vi "Actor Core.vi"(8 "error in":errorcluster, 11 "PAS Actor in":refnum<class "PAS Actor.lvclass">) -> (0 "error out":errorcluster, 3 "Actor out":refnum<class "Actor.lvclass">)   [LabVIEW 2013, in "PAS Actor.lvclass"]
doc: "(<B>Filename</B>: Actor Framework.lvlib:Actor.lvclass:Actor Core.vi)\n\nReceives messages to the actor, reacts to them, and initiates any error handling that may shut the actor down.\n\nDescendant classes may override this VI to append parallel tasks for the actor to complete while it handles messages. Overrides use the Call Parent Method node."
uses:
  PAS Actor.lvclass
  <vilib>/ActorFramework/Actor/Actor.lvclass
  PAS Actor.lvclass/PAS Actor.ctl
  <vilib>/Utility/error.llb/DialogType.ctl
  Main/PAS.lvclass
  Instrument/state.ctl
  Commands/Command.lvclass
  Instrument/Instrument.lvclass
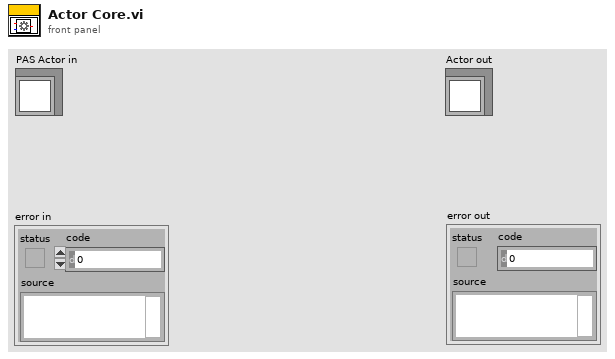
[diagram p1: front panel]
types:
  T1 = typedef "Instrument.lvclass/state.ctl" = enum8{"Configure", "Acquire", "Wait", "Quit", "Handle Error", "NOOP"}
  T2 = typedef "DialogType.ctl" = u16
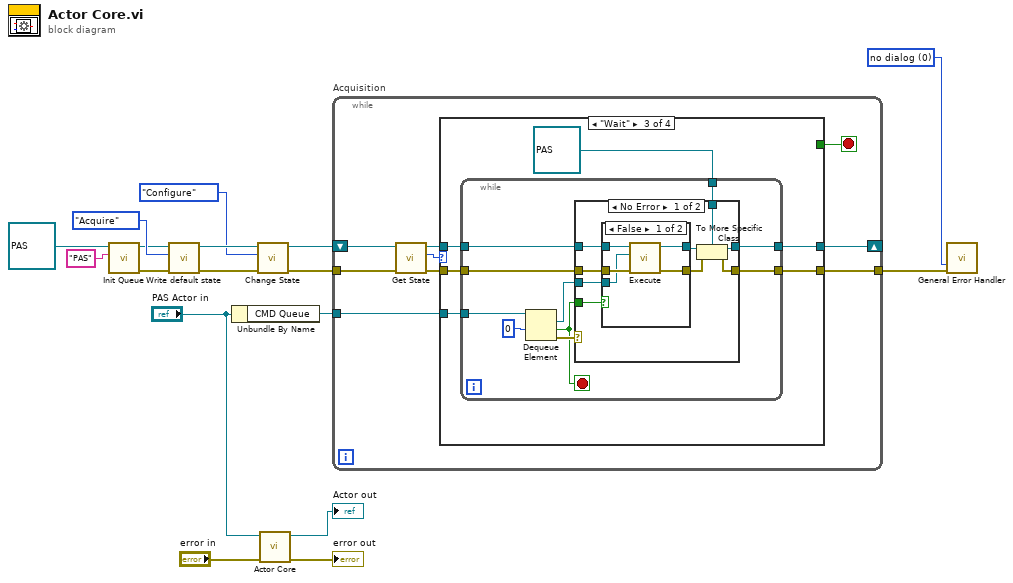
[diagram p0: block diagram]
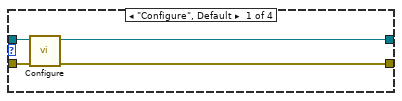
[diagram p2: hidden frame]
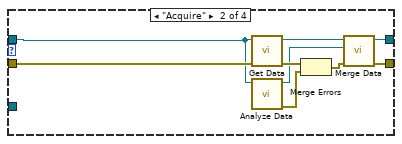
[diagram p3: hidden frame]
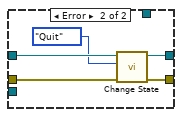
[diagram p5: hidden frame]
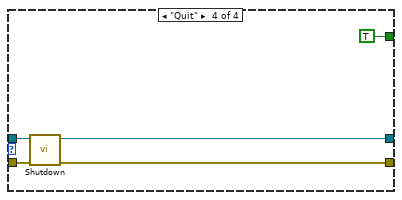
[diagram p6: hidden frame]
diagram:
  w13 = T2 0 items=["no dialog", "OK message", "continue or stop message", "OK message + warnings", "continue/stop + warnings"] ("type of dialog (OK msg:1)")
  n1 = call "Init Queue.vi"("queue_name"="PAS", "Instrument in"=refnum<class "PAS.lvclass"> refnum ("PAS")) -> ("error out"=w3:errorcluster, "Instrument out"=w4:refnum<class "PAS.lvclass">)  [unwired: 8 in]
  n2 = call "Write default state.vi"("error in (no error)"=w3, "instr state"=state."Acquire", "Instrument in"=w4) -> ("error out"=w6:errorcluster, "Instrument out"=w7:refnum<class "PAS.lvclass">)  [unwired: 7 in]
  n3 = Unbundle By Name("PAS Actor in") -> ("CMD Queue"=w11:refnum<queue>)
  n4 = call "Change State.vi"("error in"=w6, "instr state"=state."Configure", "Instrument in"=w7) -> ("error out"=w8:errorcluster, "Instrument out"=w9:refnum<class "PAS.lvclass">)  [unwired: 7 in]
  n5 = call-parent "Actor Core.vi"("error in"="error in", "Actor in"="PAS Actor in") -> ("error out"=→"error out":errorcluster, "Actor out"=→"Actor out":refnum<class "Actor.lvclass">)  [unwired: 8 in]
  n6 = while "Acquisition" {
    tunnel: w8 -> [w26]
    shift-right: [w20] -> _
    shift-left: w9 -> [w24]
    tunnel: [w19] -> w14
    tunnel: w11 -> [w18]
    stop <- w21 stop-if-true
    n7 = call "Get State.vi"("error in"=w26, "Instrument in"=w24) -> ("error out"=w22:errorcluster, "default state"=w25:T1, "Instrument out"=w23:refnum<class "PAS.lvclass">)  [unwired: 7 in]
    n8 = case shown="\"Wait\"" w25 {
      tunnel: w23 -> [w30 w38 w44 w80]
      tunnel: w22 -> [w29 w39 w42 w79]
      tunnel: [_ _ _ TRUE] -> w21
      tunnel: [w28 w34 w43 w78] -> w20
      tunnel: [w27 w32 w41 w77] -> w19
      tunnel: w18 -> [_ _ w45 _]
      frame "Configure", Default {
        n9 = call-dynamic "Configure.vi"("error in"=w29, "PAS in"=w30) -> ("error out"=w27:errorcluster, "PAS out"=w28:refnum<class "PAS.lvclass">)  [unwired: 8 in]
      }
      frame "Acquire" {
        n10 = call-dynamic "Get Data.vi"("error in"=w39, "PAS in"=w38) -> ("error out"=w37:errorcluster, "PAS out"=w35:refnum<class "PAS.lvclass">)  [unwired: 8 in]
        n11 = call-dynamic "Analyze Data.vi"("PAS in"=w38) -> ("error out"=w36:errorcluster, "PAS out"=w31:refnum<class "PAS.lvclass">)  [unwired: 9 in]
        n12 = Merge Errors(w37, w36) -> (w33:errorcluster)
        n13 = call-dynamic "Merge Data.vi"("error in"=w33, "Analyzed"=w31, "Acquired"=w35) -> ("error out"=w32:errorcluster, "PAS out"=w34:refnum<class "PAS.lvclass">)  [unwired: 7 in]
      }
      frame "Wait" {
        n14 = while {
          tunnel: w45 -> [w55]
          tunnel: w44 -> [w54]
          tunnel: [w53] -> w43
          tunnel: w42 -> [w52]
          tunnel: [w51] -> w41
          tunnel: refnum<class "PAS.lvclass"> refnum ("PAS") -> [w46]
          stop <- w48 stop-if-true
          n15 = Dequeue Element(queue=w55, timeout in ms (-1)=0) -> (element=w47:refnum<class "Command.lvclass">, timed out?=w48:bool, error out=w49:errorcluster)  [unwired: 1 in, 1 out]
          n16 = case shown="No Error" w49 {
            tunnel: w54 -> [w64 w76]
            tunnel: [w58 w74] -> w53
            tunnel: w52 -> [w63 w75]
            tunnel: [w56 w73] -> w51
            tunnel: w48 -> [w62 _]
            tunnel: w47 -> [w61 _]
            tunnel: w46 -> [w57 _]
            frame No Error {
              n17 = case shown="False" w62 {
                tunnel: w64 -> [w69 w71]
                tunnel: [w68 w71] -> w59
                tunnel: w63 -> [w67 w70]
                tunnel: [w66 w70] -> w60
                tunnel: w61 -> [w65 _]
                frame False {
                  n18 = call-dynamic "Execute.vi"("error in"=w67, "Command in"=w65, "Instrument In"=w69) -> ("error out"=w66:errorcluster, "Instrument Out"=w68:refnum<class "Instrument.lvclass">)  [unwired: 7 in]
                }
                frame True {
                }
              }
              n19 = To More Specific Class(target class=w57, reference=w59, error in=w60) -> (specific class reference=w58:refnum<class "PAS.lvclass">, error out=w56:errorcluster)
            }
            frame Error {
              n20 = call "Change State.vi"("error in"=w75, "instr state"=state."Quit", "Instrument in"=w76) -> ("error out"=w73:errorcluster, "Instrument out"=w74:refnum<class "PAS.lvclass">)  [unwired: 7 in]
            }
          }
        }
      }
      frame "Quit" {
        n21 = call-dynamic "Shutdown.vi"("error in"=w79, "PAS in"=w80) -> ("error out"=w77:errorcluster, "PAS out"=w78:refnum<class "PAS.lvclass">)  [unwired: 8 in]
      }
    }
  }
  n22 = call <vilib>:"General Error Handler.vi"("type of dialog (OK msg:1)"=w13, "error in (no error)"=w14) -> ()  [unwired: 9 in, 5 out]
